vi "8-1.vi"() -> ()   [LabVIEW 2022 SP3, in "AoC22.lvlib"]
uses:
  AoC22.lvlib
  Tree.ctl
  <vilib>/IlluminatedG/lv-stream/Stream.lvlib
panel:
  out "sum":i16
  out "Array":T1[][](array[typedef])
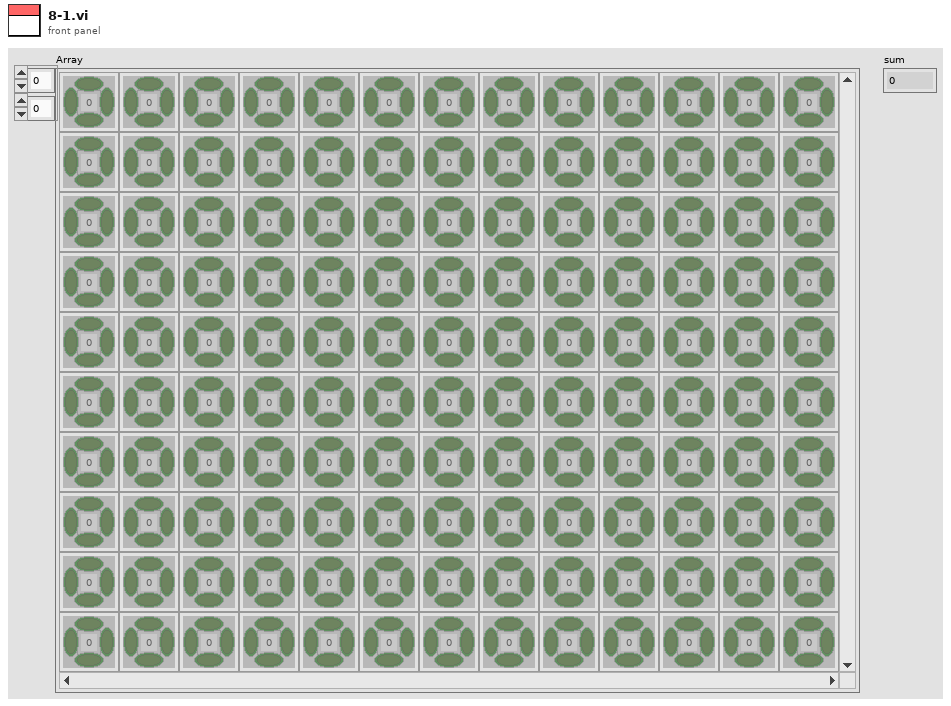
[diagram p1: front panel]
types:
  T1 = typedef "AoC22.lvlib/Tree.ctl" = cluster{"Height":i32, "Up":bool, "Left":bool, "Down":bool, "Right":bool}
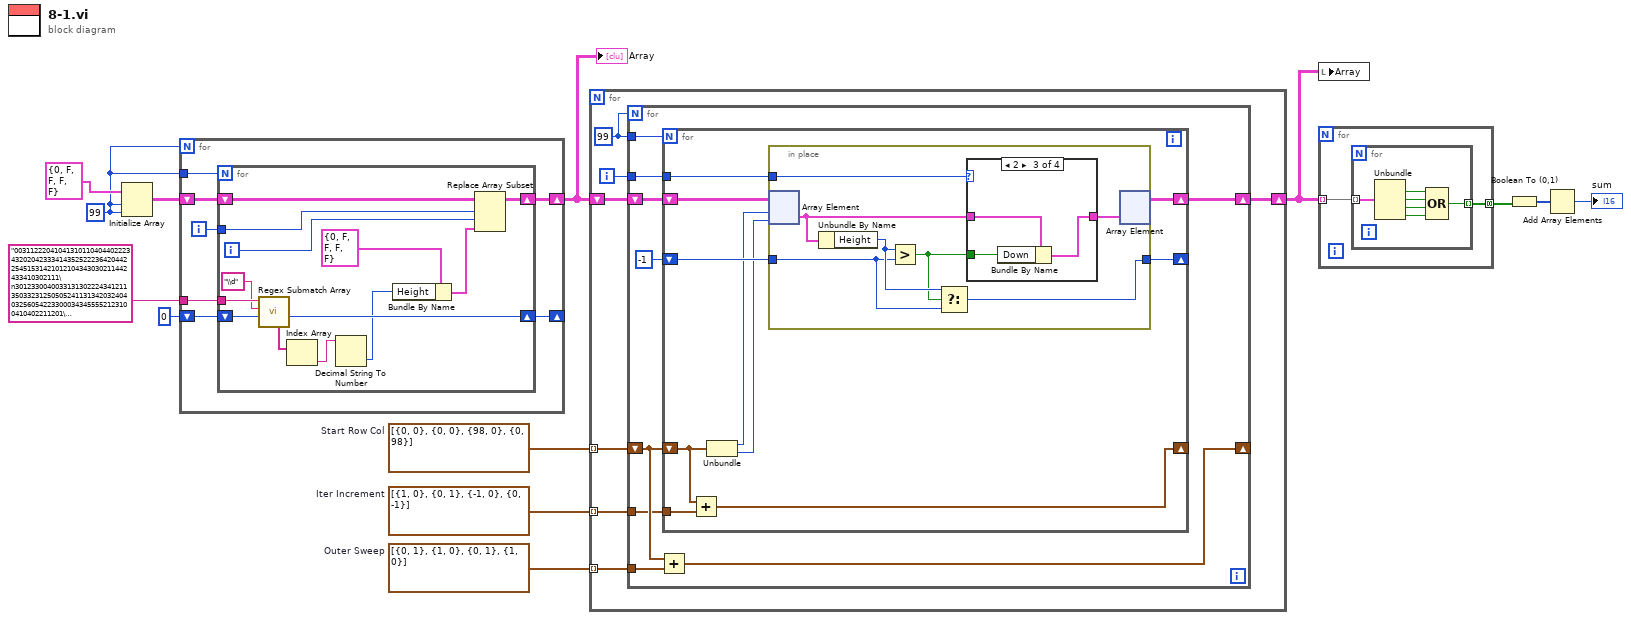
[diagram p0: block diagram]
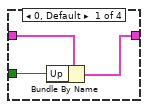
[diagram p2: hidden frame]
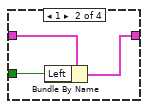
[diagram p3: hidden frame]
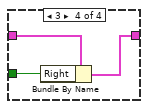
[diagram p4: hidden frame]
diagram:
  w5 = cluster{i32, i32}[] [{0, 1}, {1, 0}, {0, 1}, {1, 0}]  # Outer Sweep
  w7 = cluster{i32, i32}[] [{0, 0}, {0, 0}, {98, 0}, {0, 98}]  # Start Row Col
  w6 = cluster{i32, i32}[] [{1, 0}, {0, 1}, {-1, 0}, {0, -1}]  # Iter Increment
  w11 = 99 ("dimension size")
  n1 = Initialize Array(T1 {"Height"=0, "Up"=FALSE, "Left"=FALSE, "Down"=FALSE, "Right"=FALSE} ("Tree"), w11, w11) -> (w12:T1[][])
  n2 = for {
    N: w11 -> [_]
    shift-right: [w17] -> w8
    shift-left: w12 -> [w20]
    tunnel: w11 -> [w19]
    tunnel: "003112220410413101104044022234320204233341435252223642044225451531421012104343030211442433410302111\n301233004003313130222434121135033231250505241131342032404032560542233000343455552123100410402211201\n111301041221333142533352050250154136146324550411565615444115604102531135302000320033233340431313123\n011312210420442043155233305201305643445224334303310253225205601265233454400214114322131420224022313\n130102441231200141254202121022423405224443210463250415204410624313613034320040015223211432442333110\n133121132322223054104323242043651144066341346000104210124535555236324451132555525220523220023202433\n..." -> [w16]
    shift-right: [w15] -> _
    shift-left: 0 ("offset past match") -> [w14]
    i -> [w18]
    n3 = for {
      N: w19 -> [_]
      shift-right: [w32] -> w17
      shift-left: w20 -> [w33]
      tunnel: w18 -> [w30]
      tunnel: w16 -> [w29]
      shift-right: [w27] -> w15
      shift-left: w14 -> [w26]
      i -> [w31]
      n4 = call <vilib>:"Regex Submatch Array.vi"("offset (0)"=w26, "regular expression"="\\d", "string"=w29) -> ("offset past match"=w27:i32, "matches"=w25:string[])  [unwired: 6 in, 1 out]
      n5 = Index Array(array=w25) -> (element=w24:string)  [unwired: 1 in]
      n6 = Decimal String To Number(string=w24) -> (number=w21:i32)  [unwired: 2 in, 1 out]
      n7 = Bundle By Name(cluster=T1 {"Height"=0, "Up"=FALSE, "Left"=FALSE, "Down"=FALSE, "Right"=FALSE} ("new element/subarray"), "Height"=w21) -> (w22:T1)
      n8 = Replace Array Subset(array=w33, new element=w22, index (row)=w30, index (col)=w31) -> (w32:T1[][])
    }
  }
  "Array" <- w8
  n9 = for {
    shift-right: [w35] -> w4
    shift-left: w8 -> [w40]
    tunnel: w7 -> [w39] mode=indexing
    tunnel: w6 -> [w38] mode=indexing
    tunnel: w5 -> [w37] mode=indexing
    i -> [w34]
    w36 = 99
    n10 = for {
      N: w36 -> [_]
      shift-right: [w47] -> w35
      shift-left: w40 -> [w48]
      shift-right: [w44] -> _
      shift-left: w39 -> [w45]
      tunnel: w38 -> [w43]
      tunnel: w37 -> [w46]
      tunnel: w36 -> [w49]
      tunnel: w34 -> [w41]
      n11 = Add(x=w45, y=w46) -> (x+y=w44:cluster{i32, i32})
      n12 = for {
        N: w49 -> [_]
        shift-right: [w52] -> w47
        shift-left: w48 -> [w55]
        shift-right: [w58] -> _
        shift-left: w45 -> [w57]
        tunnel: w43 -> [w59]
        shift-right: [w53] -> _
        shift-left: -1 -> [w54]
        tunnel: w41 -> [w56]
        n13 = Add(x=w57, y=w59) -> (x+y=w58:cluster{i32, i32})
        n14 = Unbundle(w57) -> (w51:i32, w50:i32)
        n15 = in-place {
          in-place-border: w56 -> [w62]
          in-place-border: w54 -> [w65]
          in-place-border: [w64] -> w53
          n16 = in-place-array #1(w55, w51, w50) -> (w63:T1)
          n17 = Unbundle By Name(w63) -> ("Height"=w66:i32)
          n18 = Greater?(x=w66, y=w65) -> (0:w61:bool)
          n19 = Select(t=w66, s=w61, f=w65) -> (s? t:f=w64:i32)
          n20 = case shown="2" w62 {
            tunnel: w63 -> [w69 w72 w75 w78]
            tunnel: w61 -> [w68 w71 w74 w77]
            tunnel: [w67 w70 w73 w76] -> w60
            frame 0, Default {
              n21 = Bundle By Name(cluster=w69, "Up"=w68) -> (w67:T1)
            }
            frame 1 {
              n22 = Bundle By Name(cluster=w72, "Left"=w71) -> (w70:T1)
            }
            frame 2 {
              n23 = Bundle By Name(cluster=w75, "Down"=w74) -> (w73:T1)
            }
            frame 3 {
              n24 = Bundle By Name(cluster=w78, "Right"=w77) -> (w76:T1)
            }
          }
          n25 = in-place-array #1(w60) -> (w52:T1[][])  [unwired: 2 out]
        }
      }
    }
  }
  n26 = local write "Array"(w4) -> ()
  n27 = for {
    tunnel: w4 -> [w80] mode=indexing
    tunnel: [w79] -> w3 mode=concatenating
    n28 = for {
      tunnel: w80 -> [w86] mode=indexing
      tunnel: [w81] -> w79 mode=indexing
      n29 = Unbundle(w86) -> ("Up"=w85:bool, "Left"=w84:bool, "Down"=w83:bool, "Right"=w82:bool)  [unwired: 1 out]
      n30 = Compound Arithmetic op=OR(w85, w84, w83, w82) -> (w81:bool)
    }
  }
  n31 = Boolean To (0,1)(Boolean=w3) -> (0, 1=w2:i16[])
  n32 = Add Array Elements(numeric array=w2) -> (sum=→"sum":i16)
